vi "LWXPS_PositionerCompensationFrequencyNotchsSet.vi"(0 "Notch Bandwidth 1":dbl, 1 "Notch Gain 1":dbl, 2 "Notch Frequency 2":dbl, 3 "Notch Bandwidth 2":dbl, 4 "Notch Gain 2":dbl, 5 "Notch Frequency 3":dbl, 6 "Notch Frequency 1":dbl, 7 "Notch Bandwidth 3":dbl, 8 "Positioner Name":string, 9 "Notch Gain 3":dbl, 10 "XPS Reference IN":refnum<k24>, 11 "LabVIEW error IN":errorcluster) -> (14 "XPS Reference OUT":refnum<k24>, 15 "Returned error code":i32, 16 "XPS Error String":string, 19 "LabVIEW error OUT":errorcluster)   [LabVIEW 2014]
uses:
  D:/XPSQ8_LabView_Library/Development/Source/Dll/Newport.XPS.CommandInterface.dll
  Dll/Newport.XPS.CommandInterface.dll
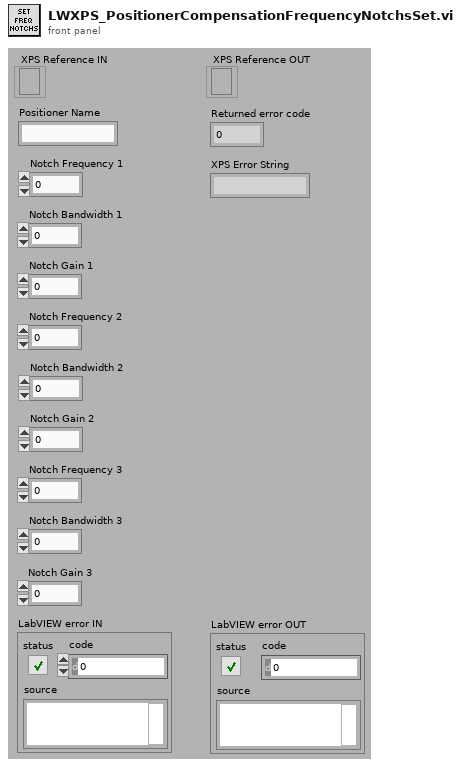
[diagram p1: front panel]
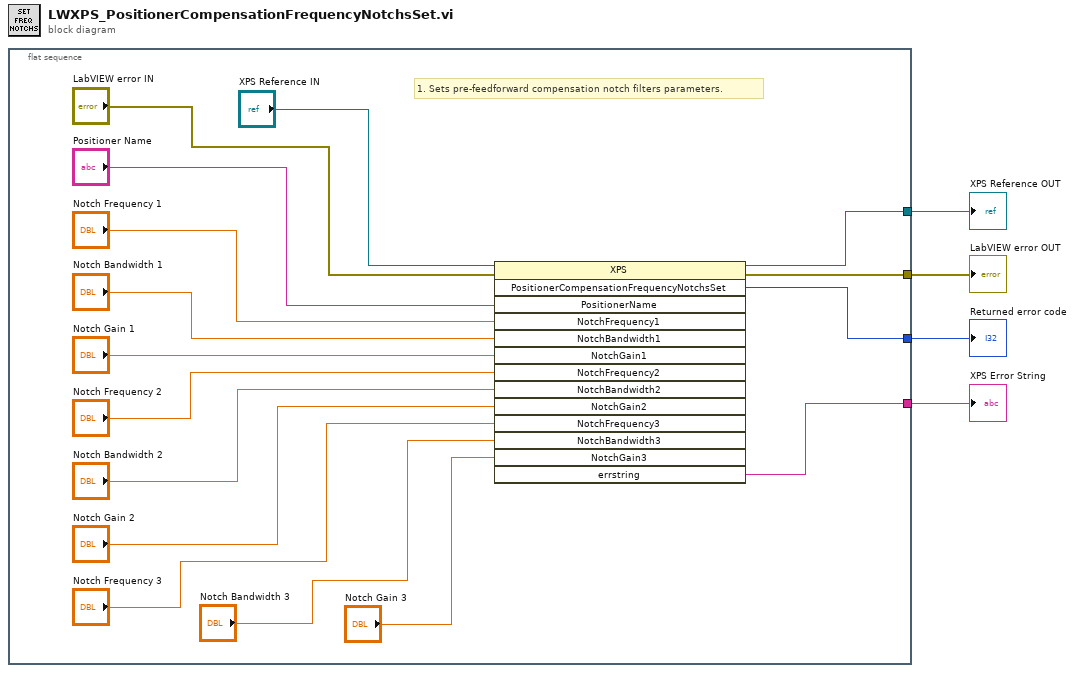
[diagram p0: block diagram]
diagram:
  n1 = flat-sequence {
    tunnel: [w18] -> w4
    tunnel: [w17] -> w3
    tunnel: [w19] -> w2
    tunnel: [w13] -> w1
    frame #0 {
      # "1. Sets pre-feedforward compensation notch filters parameters."
      n2 = invoke class="XPS" method="PositionerCompensationFrequencyNotchsSet"(reference="XPS Reference IN", error in="LabVIEW error IN", "PositionerName"="Positioner Name", "NotchFrequency1"="Notch Frequency 1", "NotchBandwidth1"="Notch Bandwidth 1", "NotchGain1"="Notch Gain 1", "NotchFrequency2"="Notch Frequency 2", "NotchBandwidth2"="Notch Bandwidth 2", "NotchGain2"="Notch Gain 2", "NotchFrequency3"="Notch Frequency 3", "NotchBandwidth3"="Notch Bandwidth 3", "NotchGain3"="Notch Gain 3") -> (reference out=w18:refnum<k24>, error out=w17:errorcluster, "PositionerCompensationFrequencyNotchsSet"=w19:i32, "errstring"=w13:string)  [unwired: 2 in, 10 out]
    }
  }
  "XPS Error String" <- w1
  "XPS Reference OUT" <- w4
  "LabVIEW error OUT" <- w3
  "Returned error code" <- w2
